vi "PH_SHS_Analysis.PC Read Cali Data.vi"(0 "i ref in":refnum<vi>, 2 "Cali Data File":path, 5 "error in (no error)":errorcluster) -> (14 "i ref out":refnum<vi>, 19 "error out":errorcluster)   [LabVIEW 2014, in "PH_SHS_Analysis.lvlib"]
doc: "This VI reads the calibration data file and sets the own attributes."
uses:
  PH_SHS_Analysis.lvlib
  PH_SHS_Analysis_Calibrator/PH_SHS_Analysis_Calibrator.lvlib
  User/Eisenbarth/SHS_v4/SHS_Analysis/SHS_Analysis.lvlib
  PH_Img_BaseClass/PH_Img_BaseClass.lvlib
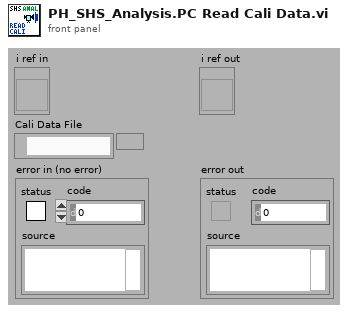
[diagram p1: front panel]
types:
  T1 = typedef "PH_SHS_Analysis_Calibrator.lvlib/PH_SHS_Analysis_Calibrator.Analysis Calibration Data.ctl" = cluster{"Date":string, "Time":string, "Cam Settings":cluster{"Cam ID":string, "Gain":dbl, "Brightness":dbl, "Shutter":dbl, "Cam Error":bool, "Mode":i32}, "SHS Reference Result":T2, "Pixel Size":dbl, "MLA Pitch":dbl, "Method":enum16{"automatic", "manual"}, "Calibration Data calculated":bool, "No Problems at calculation?":bool, "error out":errorcluster}
  T2 = typedef "SHS_Common.lvlib/SHSReference.ctl" = cluster{"Reference":T3[][], "Lens Array Pitch [px]":dbl}
  T3 = typedef "SHS_Common.lvlib/ReferencePoint.ctl" = cluster{"Rect":T4, "Point":T5}
  T4 = typedef "SHS_Common.lvlib/Rectangle.ctl" = cluster{"Left":i32, "Top":i32, "Right":i32, "Bottom":i32}
  T5 = typedef "SHS_Common.lvlib/Point.ctl" = cluster{"x":dbl, "y":dbl, "valid?":bool, "weight":dbl}
  T6 = typedef "PH_Img_BaseClass.lvlib/PH_Img_BaseClass.i attribute.ctl" = cluster{"GUI Refs":T7, "Timeout Image [ms]":i32, "Default Periodic Period [ms]":i32, "Camera":cluster{"Instancename":string, "Notifier":refnum<notifier>}, "Palette":T8, "Cam Settings":cluster{"Cam ID":string, "Gain":dbl, "Brightness":dbl, "Shutter":dbl, "Cam Info Failure":bool, "Mode":i32}}
  T7 = typedef "PH_Img_BaseClass.lvlib/PH_Img_BaseClass.GUI Refs.ctl" = cluster{"Timeout":refnum<vi>, "Image":refnum<vi>, "Palette":refnum<vi>, "Timeout Set":refnum<vi>}
  T8 = typedef "PH_Img_BaseClass.lvlib/PH_Img_BaseClass.Palette.ctl" = i32
  T9 = typedef "PH_SHS_Analysis.lvlib/PH_SHS_Analysis.i attribute.ctl" = cluster{"GUI Refs":cluster{"Delete":refnum<vi>, "Global On":refnum<vi>, "Cam Source":refnum<vi>, "Calibration Data File":refnum<vi>, "Calibration status":refnum<vi>, "Show overlay":refnum<vi>, "SHS Device Config":refnum<vi>, "Result":refnum<vi>, "Consider Tilt":refnum<vi>, "Working Reference":refnum<vi>, "Remove Tilt":refnum<vi>, "Take Cali  Reference":refnum<vi>, "Publishing Data Status":refnum<vi>, "Calibration Data":refnum<vi>}, "Calibration":cluster{"Status":T10, "Data":T1, "File":path}, "Result":T11, "Image":T14, "SHS Device Config":T15, "Show Overlay":bool, "GradientZernikeMatrix":dbl[][], "Consider Tilt":bool, "Working Reference":T2, "Zernicke Service ID":i32, "PSDB Image":T14}
  T10 = typedef "PH_StatusHandler.lvlib/PH_StatusHandler.Status.ctl" = i16
  T11 = typedef "PH_SHS_Analysis.lvlib/PH_SHS_Analysis.Result.ctl" = cluster{"Time Stamp":timestamp, "Zernike Coefficients":T12, "PtV [lambda]":dbl, "Shifts":T13, "Measurement Quality":cluster{dbl, dbl, dbl}, "Measurement valid?":bool}
  T12 = typedef "PH_SHS_Analysis.lvlib/PH_SHS_Analysis.Zernike Coefficients.ctl" = cluster{"Tilt x":dbl, "Tilt y":dbl, "Defocus":dbl, "Astig 0°":dbl, "Astig 45°":dbl, "Coma x":dbl, "Coma y":dbl, "Spherical":dbl, "Trefoil 0°":dbl, "Trefoil 30°":dbl, "2nd Astig 0°":dbl, "2nd Astig 45°":dbl, "2nd Coma x":dbl, "2nd Coma y":dbl, "2nd Spherical":dbl}
  T13 = typedef "SHS_Common.lvlib/Shifts.ctl" = T5[][]
  T14 = typedef "IMAQ Image.ctl" = refnum<image>
  T15 = typedef "SHS_Analysis.lvlib/SHS_DeviceConfig.ctl" = cluster{"focal length [m]":dbl, "pixel size [m/px]":dbl, "wavelength [m]":dbl}
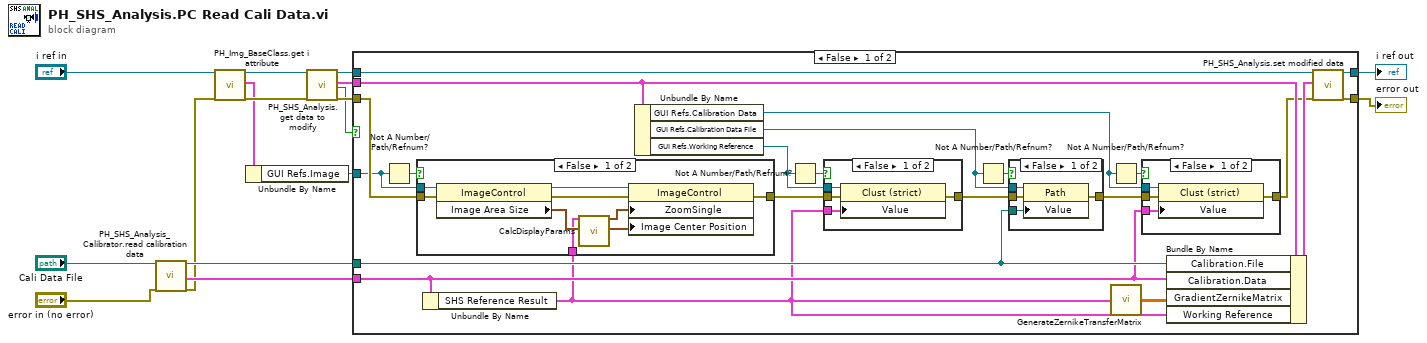
[diagram p0: block diagram]
diagram:
  n1 = call "PH_SHS_Analysis_Calibrator.read calibration data.vi"("file in"="Cali Data File", "error in (no error)"="error in (no error)") -> ("file out"=w7:path, "SHS Analysis Calibration Data"=w9:T1, "error out"=w3:errorcluster)  [unwired: 15 in]
  n2 = call "PH_Img_BaseClass.get i attribute.vi"("i ref in"="i ref in", "error in (no error)"=w3) -> ("i ref out"=w5:refnum<vi>, "i attribute"=w2:T6, "error out"=w4:errorcluster)  [unwired: 15 in]
  n3 = Unbundle By Name(w2) -> ("GUI Refs.Image"=w1:refnum<vi>)
  n4 = call "PH_SHS_Analysis.get data to modify.vi"("i ref in"=w5, "error in (no error)"=w4) -> ("i ref out"=w15:refnum<vi>, "i attribute"=w11:T9, "timed out"=w13:bool, "error out"=w16:errorcluster)  [unwired: 14 in]
  n5 = case shown="False" w13 {
    tunnel: w16 -> [w26 w64]
    tunnel: w15 -> [w38 w65]
    tunnel: [w37 w65] -> w14
    tunnel: [w36 w64] -> w12
    tunnel: w11 -> [w34 _]
    tunnel: w9 -> [w27 _]
    tunnel: w7 -> [w28 _]
    tunnel: w1 -> [w18 _]
    frame False {
      n6 = Not A Number/Path/Refnum?(number/path/refnum=w18) -> (NaN/Path/Refnum?=w25:bool)
      n7 = Unbundle By Name(w27) -> ("SHS Reference Result"=w20:T2)
      n8 = case shown="False" w25 {
        tunnel: w26 -> [w49 w53]
        tunnel: [w52 w53] -> w22
        tunnel: w18 -> [w47 _]
        tunnel: w20 -> [w44 _]
        frame False {
          n9 = property class="ImageControl"(reference=w47, error in=w49) -> (reference out=w46:refnum<vi>, error out=w48:errorcluster, "Image Area Size"=w45:cluster{"Width":u32, "Height":u32})
          n10 = call "CalcDisplayParams.vi"("SHS Reference"=w44, "Display Size"=w45) -> ("Zoom factor"=w51:cluster{"X":sgl, "Y":sgl}, "Center Position"=w50:cluster{"X":u32, "Y":u32})  [unwired: 16 in]
          n11 = property class="ImageControl"(reference=w46, error in=w48, "ZoomSingle"=w51, "Image Center Position"=w50) -> (error out=w52:errorcluster)  [unwired: 1 out]
        }
        frame True {
        }
      }
      n12 = Unbundle By Name(w34) -> ("GUI Refs.Calibration Data"=w32:refnum<vi>, "GUI Refs.Calibration Data File"=w29:refnum<vi>, "GUI Refs.Working Reference"=w23:refnum<vi>)
      n13 = Not A Number/Path/Refnum?(number/path/refnum=w23) -> (NaN/Path/Refnum?=w24:bool)
      n14 = case shown="False" w24 {
        tunnel: w22 -> [w42 w43]
        tunnel: [w41 w43] -> w21
        tunnel: w23 -> [w40 _]
        tunnel: w20 -> [w39 _]
        frame False {
          n15 = property class="Clust (strict)"(reference=w40, error in=w42, "Value"=w39) -> (error out=w41:errorcluster)  [unwired: 1 out]
        }
        frame True {
        }
      }
      n16 = Not A Number/Path/Refnum?(number/path/refnum=w29) -> (NaN/Path/Refnum?=w31:bool)
      n17 = case shown="False" w31 {
        tunnel: w21 -> [w57 w58]
        tunnel: [w56 w58] -> w30
        tunnel: w29 -> [w55 _]
        tunnel: w28 -> [w54 _]
        frame False {
          n18 = property class="Path"(reference=w55, error in=w57, "Value"=w54) -> (error out=w56:errorcluster)  [unwired: 1 out]
        }
        frame True {
        }
      }
      n19 = Not A Number/Path/Refnum?(number/path/refnum=w32) -> (NaN/Path/Refnum?=w33:bool)
      n20 = call "GenerateZernikeTransferMatrix.vi"("SHS Reference"=w20) -> ("TransferMatrix"=w19:dbl[][])
      n21 = case shown="False" w33 {
        tunnel: w30 -> [w62 w63]
        tunnel: [w61 w63] -> w17
        tunnel: w32 -> [w60 _]
        tunnel: w27 -> [w59 _]
        frame False {
          n22 = property class="Clust (strict)"(reference=w60, error in=w62, "Value"=w59) -> (error out=w61:errorcluster)  [unwired: 1 out]
        }
        frame True {
        }
      }
      n23 = Bundle By Name(cluster=w34, "Calibration.File"=w28, "Calibration.Data"=w27, "GradientZernikeMatrix"=w19, "Working Reference"=w20) -> (w35:T9)
      n24 = call "PH_SHS_Analysis.set modified data.vi"("i ref in"=w38, "i attribute"=w35, "error in (no error)"=w17) -> ("i ref out"=w37:refnum<vi>, "error out"=w36:errorcluster)  [unwired: 15 in]
    }
    frame True {
    }
  }
  "i ref out" <- w14
  "error out" <- w12
